vi "reset piezo to 0V.vi"(8 "error in":errorcluster) -> (0 "error out":errorcluster)   [LabVIEW 2017]
doc: "SciScan 1.2 160622"
uses:
  <vilib>/DAQmx/write.llb/DAQmx Write (Analog DBL 1Chan 1Samp).vi
  GFG/GFGbooleanGet.vi
  GFG/GFGnumericGet.vi
  <vilib>/DAQmx/create/channels.llb/DAQmx Create Channel (AO-Voltage-Basic).vi
  <vilib>/DAQmx/miscellaneous.llb/DAQmx Fill In Error Info.vi
  GFG/GFG library.lvlib
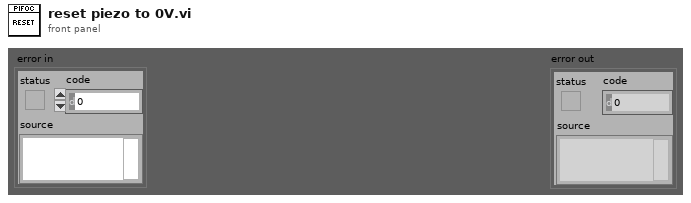
[diagram p1: front panel]
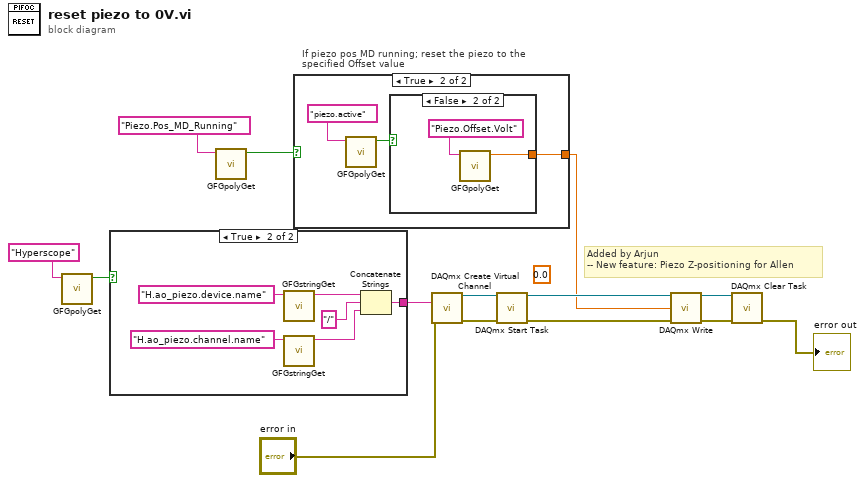
[diagram p0: block diagram]
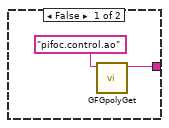
[diagram p2: hidden frame]
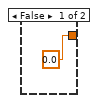
[diagram p3: hidden frame]
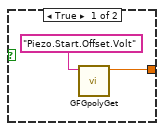
[diagram p4: hidden frame]
diagram:
  (unwired) 0.0 ("data")
  # "Added by Arjun\n-- New feature: Piezo Z-positioning for Allen"
  n1 = call-poly "GFGpolyGet.vi"("Variable Name in"="Hyperscope") -> ("Boolean Value OUT"=w1:bool)  [unwired: 9 in, 1 out]
  n2 = case shown="True" w1 {
    tunnel: [w15 w17] -> w8
    frame False {
      n3 = call-poly "GFGpolyGet.vi"("Variable Name in"="pifoc.control.ao") -> ("String"=w15:string)  [unwired: 9 in, 1 out]
    }
    frame True {
      n4 = call "GFGstringGet.vi"("Variable Name in"="H.ao_piezo.device.name") -> ("String"=w20:string)  [unwired: 9 in, 1 out]
      n5 = call "GFGstringGet.vi"("Variable Name in"="H.ao_piezo.channel.name") -> ("String"=w18:string)  [unwired: 9 in, 1 out]
      n6 = Concatenate Strings(w20, "/" ("string"), w18) -> (w17:string)
    }
  }
  n7 = call-poly "GFGpolyGet.vi"("Variable Name in"="Piezo.Pos_MD_Running") -> ("Boolean Value OUT"=w4:bool)  [unwired: 9 in, 1 out]
  n8 = case "If piezo pos MD running; reset the piezo to the specified Offset value" shown="True" w4 {
    tunnel: [0.0 ("Numeric") w26] -> w3
    frame False {
    }
    frame True {
      n9 = call-poly "GFGpolyGet.vi"("Variable Name in"="piezo.active") -> ("Boolean Value OUT"=w24:bool)  [unwired: 9 in, 1 out]
      n10 = case shown="False" w24 {
        tunnel: [w27 w29] -> w26
        frame True {
          n11 = call-poly "GFGpolyGet.vi"("Variable Name in"="Piezo.Start.Offset.Volt") -> ("Numeric"=w27:dbl)  [unwired: 8 in, 2 out]
        }
        frame False {
          n12 = call-poly "GFGpolyGet.vi"("Variable Name in"="Piezo.Offset.Volt") -> ("Numeric"=w29:dbl)  [unwired: 8 in, 2 out]
        }
      }
    }
  }
  n13 = call-poly <vilib>:"DAQmx Create Virtual Channel.vi"("physical channels"=w8, "error in"="error in") -> ("task out"=w10:refnum<k21>, "error out"=w9:errorcluster)  [unwired: 12 in]
  n14 = call <vilib>:"DAQmx Start Task.vi"("task/channels in"=w10, "error in"=w9) -> ("task out"=w12:refnum<k21>, "error out"=w14:errorcluster)  [unwired: 12 in]
  n15 = call-poly <vilib>:"DAQmx Write.vi"("task/channels in"=w12, "data"=w3, "error in"=w14) -> ("task out"=w11:refnum<k21>, "error out"=w13:errorcluster)  [unwired: 10 in, 1 out]
  n16 = call <vilib>:"DAQmx Clear Task.vi"("task in"=w11, "error in"=w13) -> ("error out"=→"error out":errorcluster)  [unwired: 13 in]
